vi "DS_transmissions.vi"(4 "start":dbl, 6 "end":dbl, 9 "xi in":dbl[](array[numeric]), 10 "wavelengths":dbl[](array[numeric]), 11 "trunc transmissions[r=wl, c=v]":dbl[][](array[numeric])) -> (0 "end (out)":dbl, 1 "start (out)":dbl, 2 "transmissions[r=wl, c=v]":dbl[][](array[numeric]), 3 "xi used":dbl[](array[numeric]))   [LabVIEW 2019]
uses:
  <vilib>/gmath/NI_Gmath.lvlib
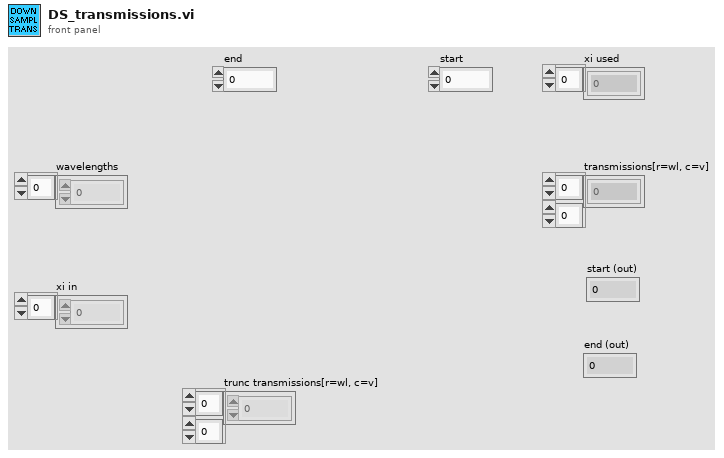
[diagram p1: front panel]
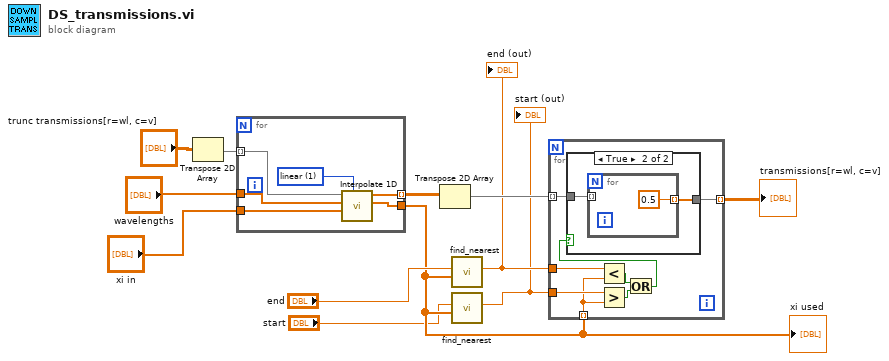
[diagram p0: block diagram]
diagram:
  n1 = Transpose 2D Array(2D array="trunc transmissions[r=wl, c=v]") -> (transposed array=w10:dbl[][])
  n2 = for {
    tunnel: w10 -> [w17] mode=indexing
    tunnel: [w15] -> w11 mode=indexing
    tunnel: "wavelengths" -> [w16]
    tunnel: "xi in" -> [w18]
    tunnel: [w13] -> w3
    w14 = 1 items=["nearest", "linear", "spline", "cubic Hermite", "Lagrange"] ("method")
    n3 = call <vilib>:"Interpolate 1D.vi"("method"=w14, "xi"=w18, "X"=w16, "Y"=w17) -> ("xi used"=w13:dbl[], "yi"=w15:dbl[])  [unwired: 5 in, 1 out]
  }
  "xi used" <- w3
  n4 = Transpose 2D Array(2D array=w11) -> (transposed array=w7:dbl[][])
  n5 = call "find_nearest.vi"("Sorted Array (<)"=w3, "Key"="end") -> ("Nearest"=w4:dbl)  [unwired: 6 in, 3 out]
  "end (out)" <- w4
  n6 = call "find_nearest.vi"("Sorted Array (<)"=w3, "Key"="start") -> ("Nearest"=w1:dbl)  [unwired: 6 in, 3 out]
  "start (out)" <- w1
  n7 = for {
    tunnel: w4 -> [w26]
    tunnel: w1 -> [w25]
    tunnel: [w21] -> w6 mode=indexing
    tunnel: w7 -> [w20] mode=indexing
    tunnel: w3 -> [w19] mode=indexing
    n8 = Less?(x=w26, y=w19) -> (x < y?=w23:bool)
    n9 = Greater?(x=w25, y=w19) -> (0:w24:bool)
    n10 = Or(x=w23, y=w24) -> (x .or. y?=w22:bool)
    n11 = case shown="True" w22 {
      tunnel: [w27 w29] -> w21
      tunnel: w20 -> [w27 w28]
      frame False {
      }
      frame True {
        n12 = for {
          tunnel: [0.5] -> w29 mode=indexing
          tunnel: w28 -> [_] mode=indexing
        }
      }
    }
  }
  "transmissions[r=wl, c=v]" <- w6
